vi "write relay.vi"(6 "wait for reply (T)":bool=TRUE, 8 "error in":errorcluster, 9 "High/Low":bool, 10 "Line Enum":T1, 11 "Module ID":i32=-1) -> (0 "error out":errorcluster, 1 "timed out?":bool)   [LabVIEW 2025, in "USB IO.lvlib"]
doc: "Writes single relay\n\n_____\nCreated using DQMH Framework: Event Scripter 7.1.2.1547."
uses:
  USB IO.lvlib
  Classes/USB IO/Relay Line.ctl
  write relay Argument--cluster.ctl
  write relay (Reply Payload)--cluster.ctl
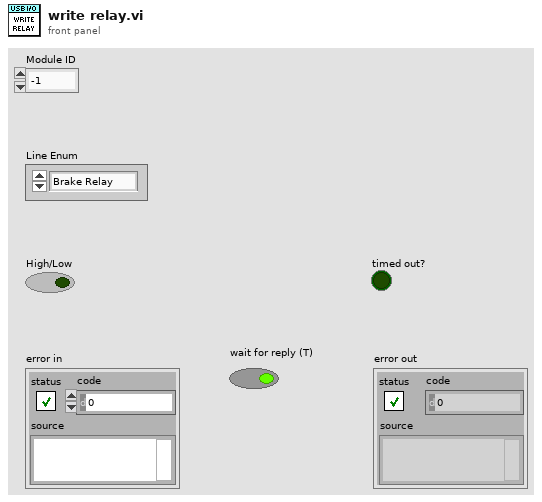
[diagram p1: front panel]
types:
  T1 = typedef "Relay Line.ctl" = enum16{"Brake Relay", "PS Relay"}
  T2 = typedef "USB IO.lvlib/write relay Argument--cluster.ctl" = cluster{"Module ID":i32, "Line Enum":T1, "High/Low":bool, "Wait Notifier":refnum<notifier>, "wait for reply":bool}
  T3 = typedef "USB IO.lvlib/Request Events--cluster.ctl" = cluster{"Stop Module":refnum<user-event>, "Show Panel":refnum<user-event>, "Hide Panel":refnum<user-event>, "Show Diagram":refnum<user-event>, "Get Module Execution Status":refnum<user-event>, "read config":refnum<user-event>, "init":refnum<user-event>, "close":refnum<user-event>, "write relay":refnum<user-event>}
  T4 = typedef "USB IO.lvlib/write relay (Reply Payload)--cluster.ctl" = cluster{"Module ID":i32, "error":errorcluster}
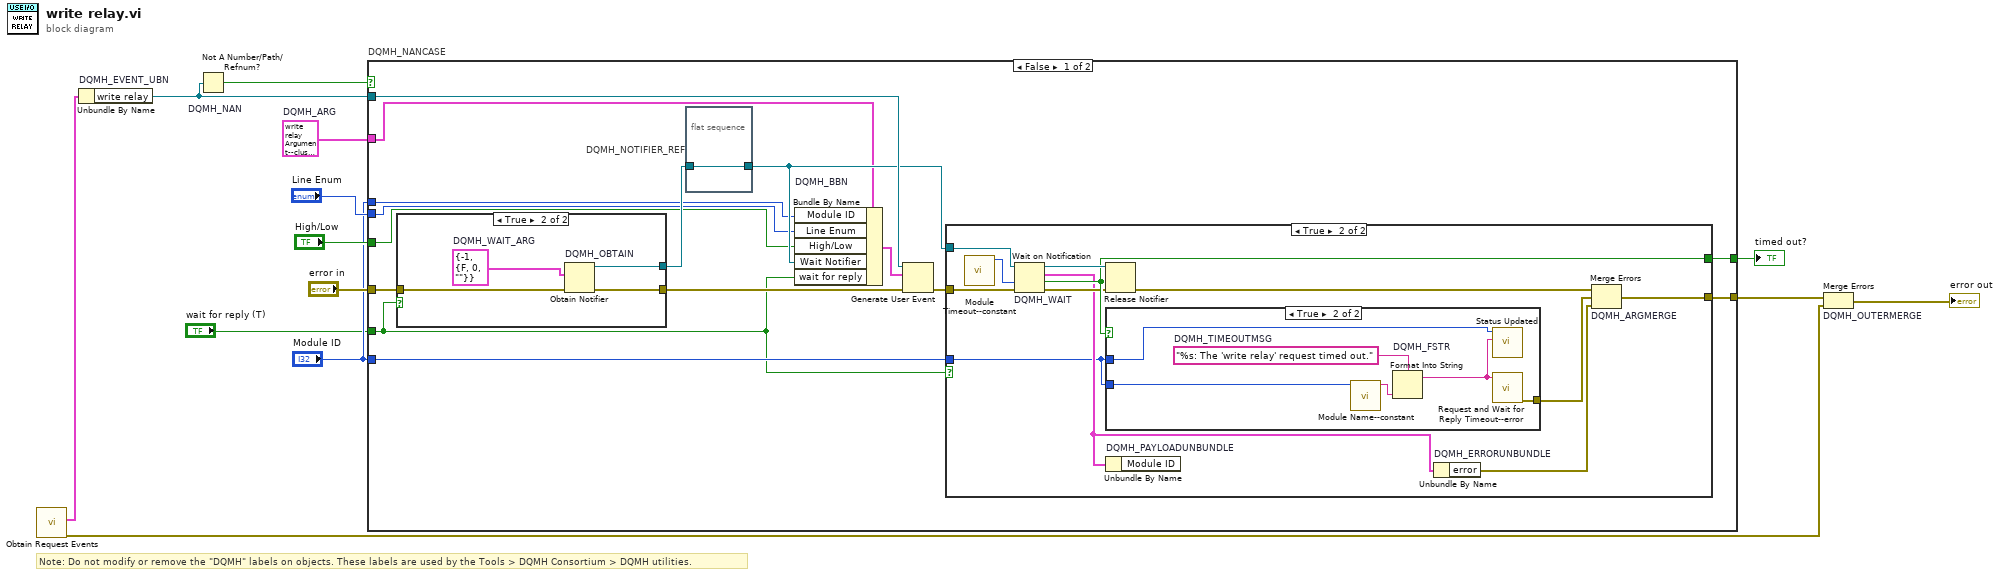
[diagram p0: block diagram]
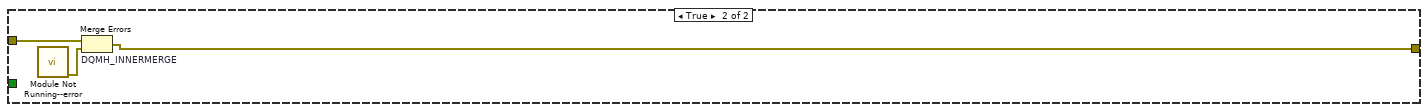
[diagram p5: hidden frame]
diagram:
  w7 = T2 {"Module ID"=-1, "Line Enum"=enum."Brake Relay", "High/Low"=FALSE, "Wait Notifier"=refnum, "wait for reply"=FALSE}  # DQMH_ARG
  # "Note: Do not modify or remove the \"DQMH\" labels on objects. These labels are used by the Tools > DQMH Consortium > DQMH utilities."
  n1 = call "Obtain Request Events.vi"() -> ("error out"=w2:errorcluster, "USB IO Request Events"=w1:T3)  [unwired: 10 in]
  n2 = Unbundle By Name "DQMH_EVENT_UBN"(w1) -> ("write relay"=w11:refnum<user-event>)
  n3 = Not A Number/Path/Refnum? "DQMH_NAN"(number/path/refnum=w11) -> (NaN/Path/Refnum?=w10:bool)
  n4 = case "DQMH_NANCASE" shown="False" w10 {
    tunnel: "error in" -> [w28 w56]
    tunnel: w11 -> [w26 _]
    tunnel: [w23 w55] -> w8
    tunnel: [w24 _] -> w9
    tunnel: w7 -> [w19 _]
    tunnel: "Module ID" -> [w18 _]
    tunnel: "Line Enum" -> [w17 _]
    tunnel: "High/Low" -> [w16 _]
    tunnel: "Module ID" -> [w15 _]
    tunnel: "wait for reply (T)" -> [w14 _]
    frame False {
      n5 = case shown="True" w14 {
        tunnel: w28 -> [w49 w53]
        tunnel: [w49 w52] -> w25
        tunnel: [_ w50] -> w21
        frame False {
        }
        frame True {
          w51 = T4 {"Module ID"=-1, "error"={"status"=FALSE, "code"=0, "source"=""}}  # DQMH_WAIT_ARG
          n6 = Obtain Notifier "DQMH_OBTAIN"(notification data type=w51, error in (no error)=w53) -> (notifier out=w50:refnum<notifier>, error out=w52:errorcluster)  [unwired: 2 in, 1 out]
        }
      }
      n7 = flat-sequence "DQMH_NOTIFIER_REF" {
        tunnel: w21 -> [w29]
        tunnel: [w29] -> w20
        frame #0 {
        }
      }
      n8 = Bundle By Name "DQMH_BBN"(cluster=w19, "Module ID"=w18, "Line Enum"=w17, "High/Low"=w16, "Wait Notifier"=w20, "wait for reply"=w14) -> (w22:T2)
      n9 = Generate User Event(user event=w26, event data cluster=w22, error in=w25) -> (error out=w27:errorcluster)  [unwired: 1 in, 1 out]
      n10 = case shown="True" w14 {
        tunnel: w27 -> [w30 w42]
        tunnel: w20 -> [_ w41]
        tunnel: [_ w39] -> w24
        tunnel: [w30 w38] -> w23
        tunnel: w15 -> [_ w31]
        frame False {
        }
        frame True {
          n11 = call "Module Timeout--constant.vi"() -> ("Module Timeout"=w32:i32)  [unwired: 11 in]
          n12 = Wait on Notification "DQMH_WAIT"(notifier=w41, timeout in ms (-1)=w32, error in (no error)=w42) -> (notifier out=w40:refnum<notifier>, notification=w33:T4, timed out?=w39:bool, error out=w37:errorcluster)  [unwired: 1 in]
          n13 = Release Notifier(notifier=w40, error in (no error)=w37) -> (error out=w36:errorcluster)  [unwired: 1 in, 2 out]
          n14 = case shown="True" w39 {
            tunnel: [_ w46] -> w34
            tunnel: w31 -> [_ w44]
            tunnel: w31 -> [_ w43]
            frame False {
            }
            frame True {
              w48 = "%s: The 'write relay' request timed out."  # DQMH_TIMEOUTMSG
              n15 = call "Module Name--constant.vi"("Module ID"=w43) -> ("Module Name"=w45:string)  [unwired: 10 in]
              n16 = Format Into String "DQMH_FSTR"(format string=w48, w45) -> (resulting string=w47:string)  [unwired: 2 in, 1 out]
              n17 = call "Status Updated.vi"("Status"=w47, "Module ID"=w44) -> ()  [unwired: 9 in, 1 out]
              n18 = call "Request and Wait for Reply Timeout--error.vi"("Error Message"=w47) -> ("error out"=w46:errorcluster)  [unwired: 10 in]
            }
          }
          n19 = Unbundle By Name "DQMH_PAYLOADUNBUNDLE"(w33) -> ()  [unwired: 1 out]
          n20 = Unbundle By Name "DQMH_ERRORUNBUNDLE"(w33) -> ("error"=w35:errorcluster)
          n21 = Merge Errors "DQMH_ARGMERGE"(w36, w34, w35) -> (w38:errorcluster)
        }
      }
    }
    frame True {
      n22 = call "Module Not Running--error.vi"() -> ("error out"=w54:errorcluster)  [unwired: 11 in]
      n23 = Merge Errors "DQMH_INNERMERGE"(w56, w54) -> (w55:errorcluster)
    }
  }
  "timed out?" <- w9
  n24 = Merge Errors "DQMH_OUTERMERGE"(w8, w2) -> (→"error out":errorcluster)
